vi "UUID.vi"() -> (3 "UUID":string)   [LabVIEW 2020]
panel:
  out "EffectiveDate":u64
  out "Effective":bool
  out "所有大写字母字符串":string
  out "MD5 message-digest":string
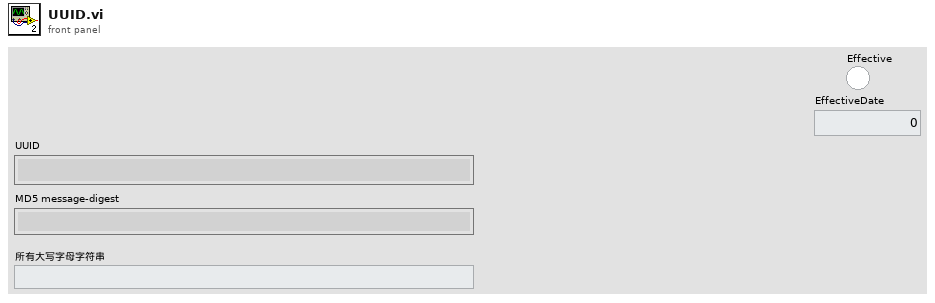
[diagram p1: front panel]
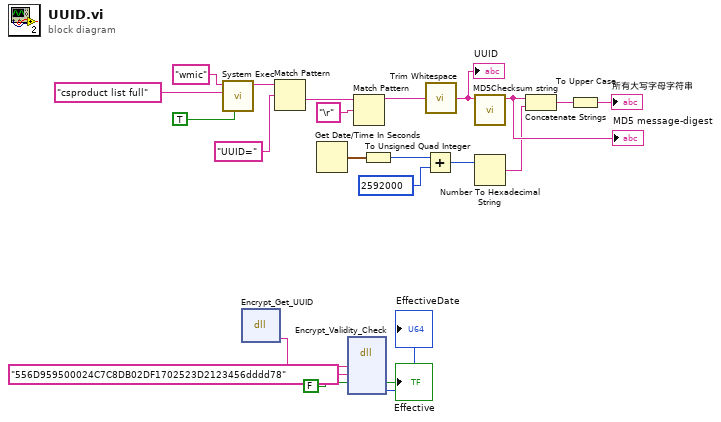
[diagram p0: block diagram]
diagram:
  n1 = call <vilib>:"System Exec.vi"("run minimized? (F)"=TRUE, "standard input"="csproduct list full", "command line"="wmic") -> ("standard output"=w19:string)  [unwired: 5 in, 3 out]
  n2 = dll-call lib="PTH2Pabs CUsersFeng项目HLCEPSbuilds020磨合台EncryptEncrypt.dll" fn="Encrypt_Get_UUID"() -> ("UUID"=w5:string)  [unwired: 5 in, 2 out]
  n3 = Match Pattern(string=w19, regular expression="UUID=" ("正则表达式")) -> (after substring=w17:string)  [unwired: 1 in, 3 out]
  n4 = Get Date/Time In Seconds() -> (seconds since 1Jan1904=w13:timestamp)
  n5 = dll-call lib="PTH2Pabs CUsersFeng项目HLCEPSbuilds020磨合台EncryptEncrypt.dll" fn="Encrypt_Validity_Check"("UUID"=w5, "KEY"="556D959500024C7C8DB02DF1702523D2123456dddd78", "Effective"=FALSE) -> ("Effective"=→"Effective":bool, "EffectiveDate"=→"EffectiveDate":u64)  [unwired: 7 in, 2 out]
  n6 = Match Pattern(string=w17, regular expression="\r" ("正则表达式")) -> (before substring=w16:string)  [unwired: 1 in, 3 out]
  n7 = To Unsigned Quad Integer(1:w13) -> (0:w12:u64)
  n8 = Add(x=w12, y=u64 2592000) -> (x+y=w10:u64)
  n9 = call <vilib>:"Trim Whitespace.vi"("string"=w16) -> ("trimmed string"=w14:string)  [unwired: 1 in]
  "UUID" <- w14
  n10 = call <vilib>:"MD5Checksum string.vi"("Message String"=w14) -> ("MD5 message-digest"=w9:string)  [unwired: 10 in]
  "MD5 message-digest" <- w9
  n11 = Number To Hexadecimal String(2:w10) -> (0:w8:string)  [unwired: 1 in]
  n12 = Concatenate Strings(w9, w8) -> (w7:string)
  n13 = To Upper Case(1:w7) -> (0:→"所有大写字母字符串":string)
